vi "PatchViewer.vi"() -> ()   [LabVIEW 2016]
uses:
  <vilib>/Utility/sysdir.llb/System Directory Type.ctl
  <vilib>/Utility/file.llb/Read From Spreadsheet File (DBL).vi
  <vilib>/Utility/file.llb/Write To Spreadsheet File (DBL).vi
  <vilib>/vision/NI_Vision_Development_Module.lvlib
  <vilib>/ptbypt/NI_PtbyPt.lvlib
panel:
  in  "Diff":dbl
  in  "REC":bool
  out "all rows":dbl[][](array[numeric])
  in  "Gamma":dbl(slide)=0.5 min=0.5 max=2.0 step=0.1 scale=0.5..2.0
  in  "Contrast":i64(slide) caption="Gain (Raw)" min=0 max=384 step=1 scale=0.0..100.0
  in  "AutoContrast":bool
  in  "AutoExposure":bool
  in  "Decrease":bool
  in  "Increase":bool
  in  "set 4":bool
  in  "set 3":bool
  in  "set 2":bool
  in  "set 1":bool
  in  "pos 4":bool
  in  "pos 3":bool
  in  "pos 2":bool
  in  "pos 1":bool
  in  "zoom 4":bool
  in  "zoom 3":bool
  in  "zoom 2":bool
  in  "zoom1":bool
  out "fps":dbl
  in  "stop":bool
  in  "Gain":dbl(slide)=1.0 min=1.0 max=4.0 scale=1.0..4.0
  in  "Exposure Time (ms)":dbl(slide)=32000.0 caption="Exposure Time" min=2000.0 max=32000.0 scale=2000.0..32000.0 scale format="%^#_3g"
  out "Image Out":T1(plugin-control)
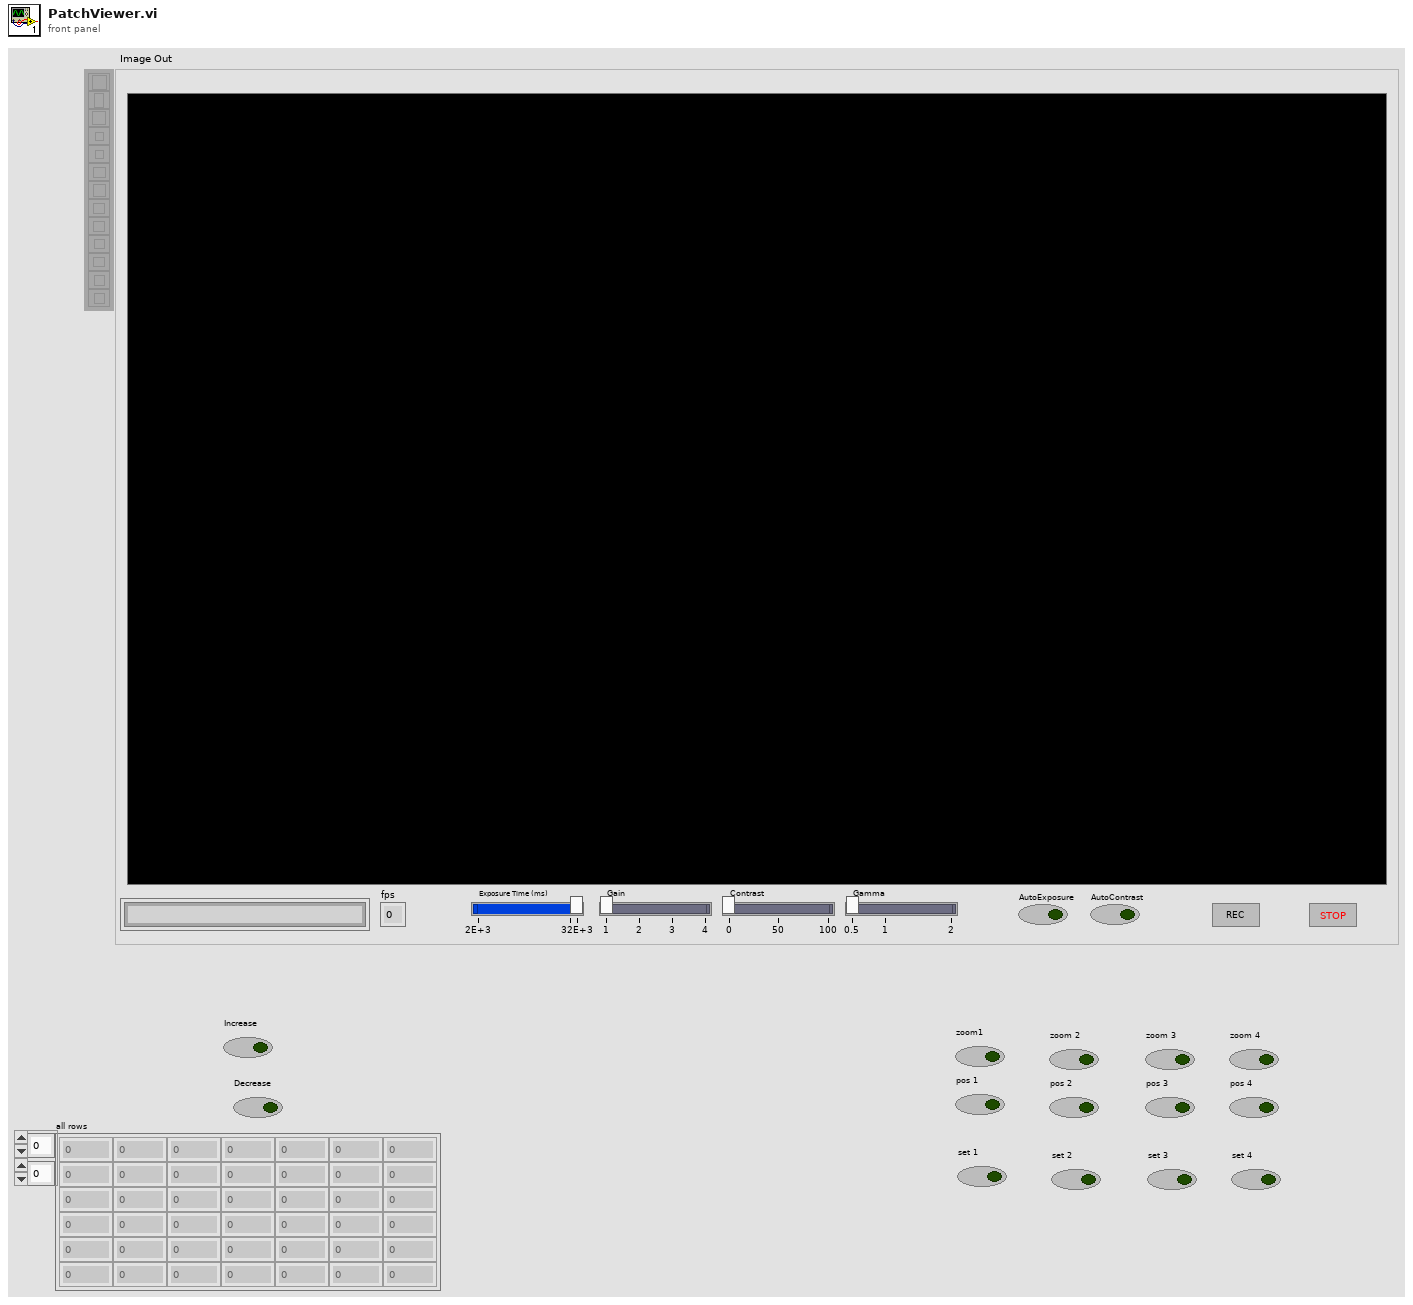
[diagram p1: front panel]
types:
  T1 = typedef "IMAQ Image.ctl" = refnum<image>
  T2 = cluster{"Brightness":sgl, "Contrast":sgl, "Gamma":sgl}
  T3 = cluster{"Mean Value":sgl, "Standard Variation":sgl, "Minimal Value":sgl, "Maximal Value":sgl, "Area (calibrated)":sgl, "Area (pixels)":u32, "%":sgl, "Calibration Valid":bool}
  T4 = typedef "System Directory Type.ctl" = i32
  T5 = typedef "IMAQ AVI2 Refnum.ctl" = refnum<k20>
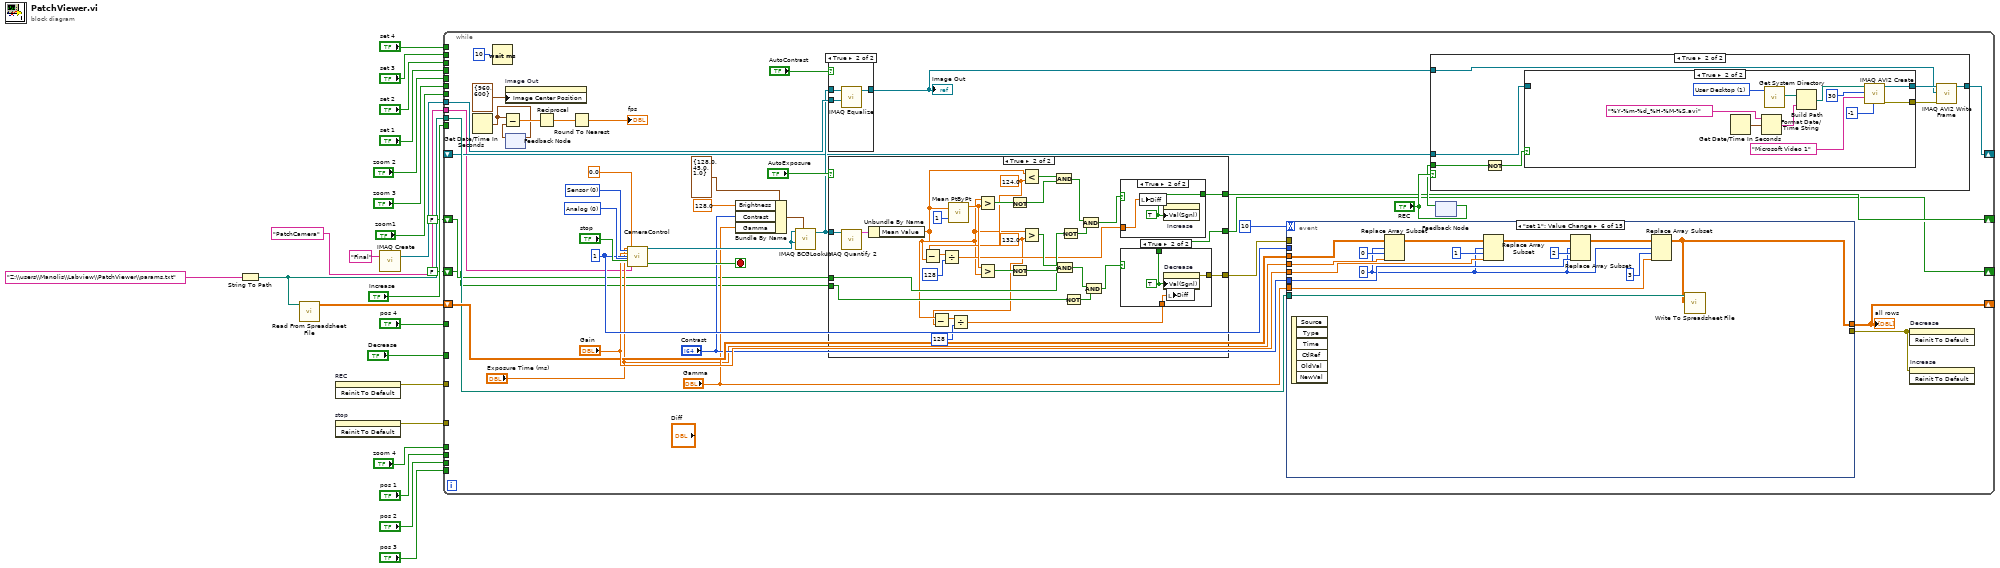
[diagram p0: block diagram]
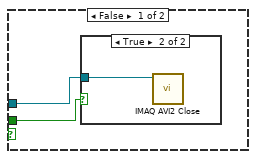
[diagram p2: hidden frame]
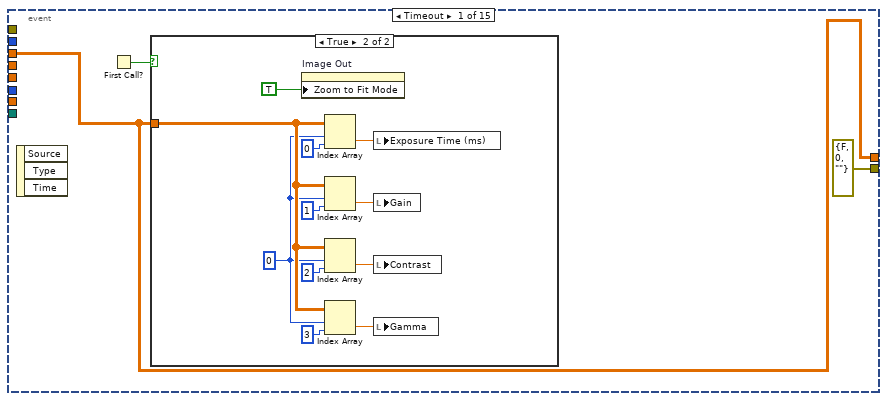
[diagram p9: hidden frame]
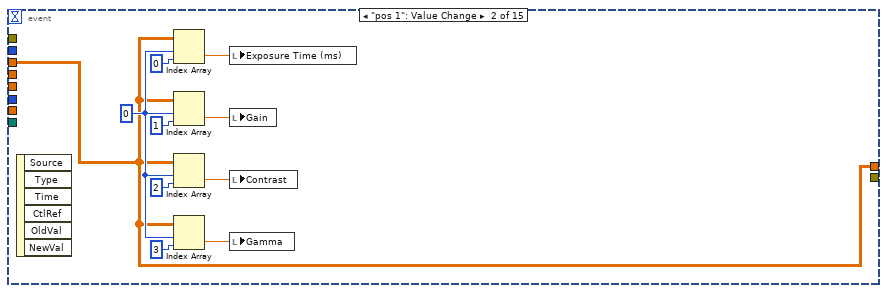
[diagram p11: hidden frame]
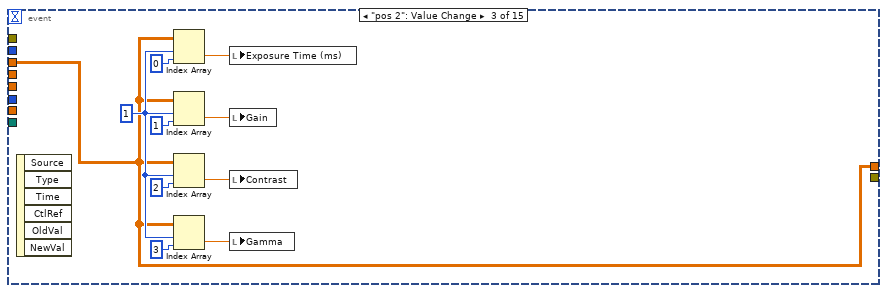
[diagram p12: hidden frame]
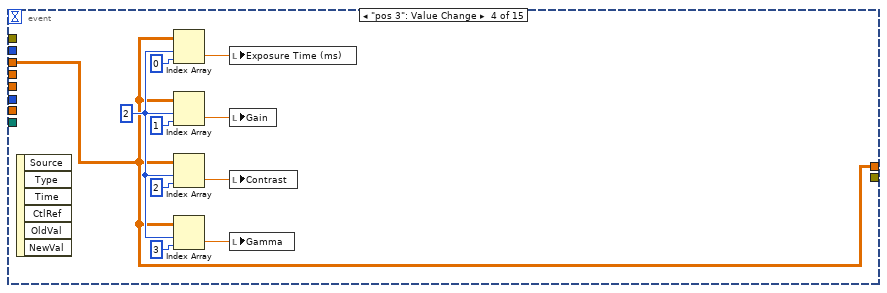
[diagram p13: hidden frame]
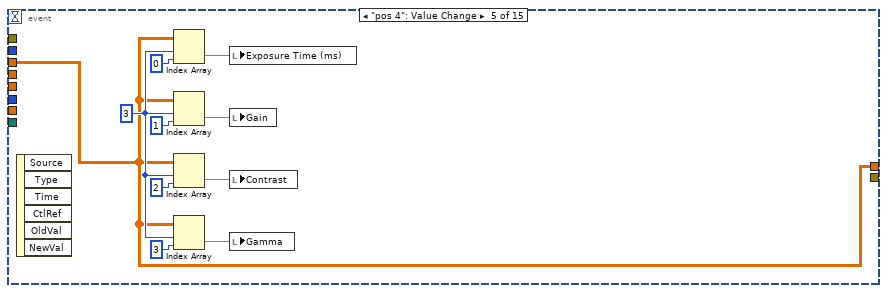
[diagram p14: hidden frame]
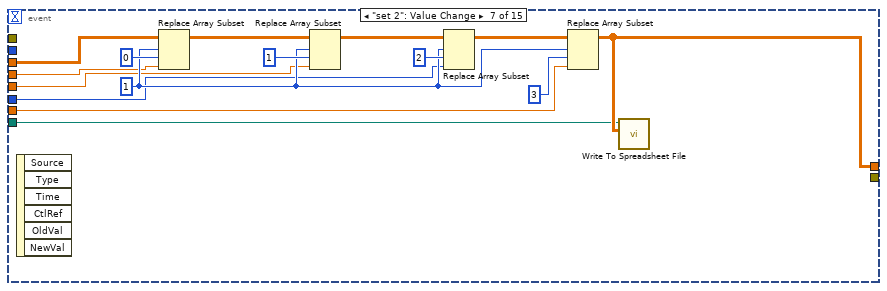
[diagram p15: hidden frame]
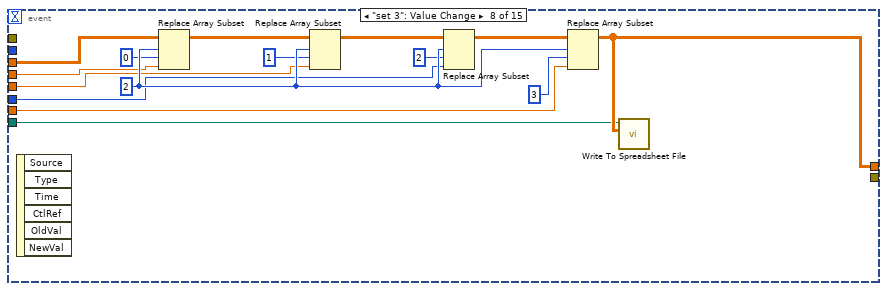
[diagram p16: hidden frame]
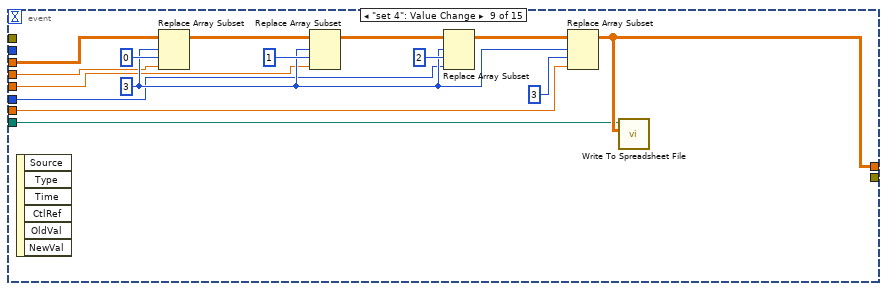
[diagram p17: hidden frame]
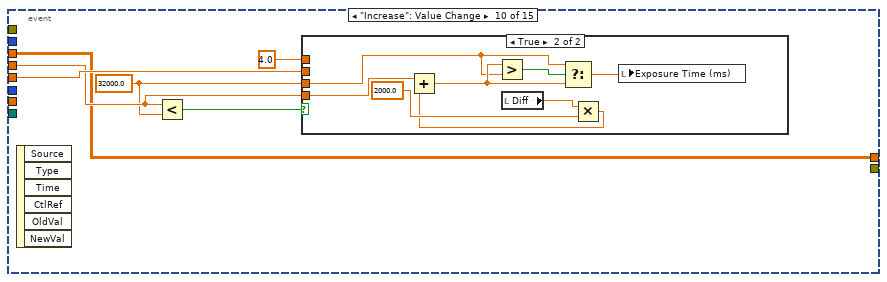
[diagram p18: hidden frame]
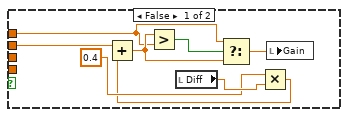
[diagram p19: hidden frame]
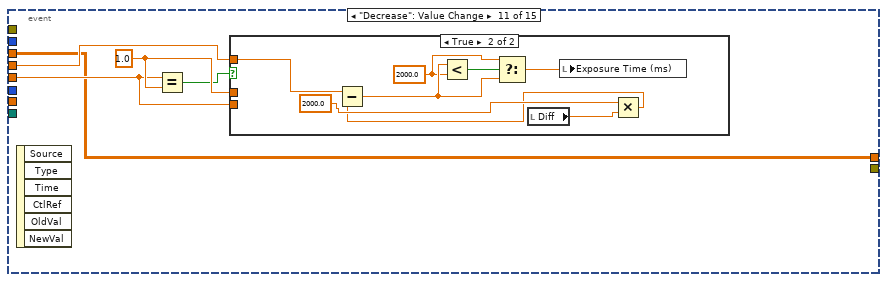
[diagram p20: hidden frame]
diagram:
  n1 = String To Path(string="Z:\\users\\Manolis\\Labview\\PatchViewer\\params.txt") -> (path=w6:path)
  n2 = call-poly <vilib>:"Read From Spreadsheet File.vi"("file path (dialog if empty)"=w6) -> ("all rows"=w7:dbl[][])  [unwired: 6 in, 4 out]
  n3 = invoke on="REC" class="Bool (strict)" method="Reinit To Default"() -> (error out=w5:errorcluster)  [unwired: 3 in, 2 out]
  n4 = invoke on="stop" class="Bool" method="Reinit To Default"() -> (error out=w4:errorcluster)  [unwired: 3 in, 2 out]
  n5 = call "IMAQ Create"("Image Name"="Final") -> ("New Image"=w9:T1)  [unwired: 4 in, 1 out]
  n6 = while {
    tunnel: "pos 4" -> [_]
    tunnel: "pos 3" -> [_]
    tunnel: "pos 2" -> [_]
    tunnel: "pos 1" -> [_]
    tunnel: "zoom1" -> [_]
    tunnel: "zoom 4" -> [_]
    tunnel: "set 4" -> [_]
    tunnel: "set 3" -> [_]
    tunnel: "set 2" -> [_]
    tunnel: "set 1" -> [_]
    tunnel: "zoom 2" -> [_]
    tunnel: "zoom 3" -> [_]
    tunnel: "Increase" -> [_]
    tunnel: "Decrease" -> [_]
    tunnel: w9 -> [w48]
    shift-right: [w45] -> _
    shift-left: w7 -> [w46]
    tunnel: w6 -> [w44]
    shift-right: [w33] -> _
    shift-left: _ -> [w32]
    tunnel: w5 -> [_]
    tunnel: w4 -> [_]
    tunnel: "PatchCamera" -> [w29]
    shift-right: [w28] -> _
    shift-left: FALSE ("Value (Signaling)") -> [w27]
    shift-right: [w26] -> _
    shift-left: FALSE ("Value (Signaling)") -> [w25]
    stop <- w65 stop-if-true
    w53 = i64 1 ("Gain (Raw)")
    w63 = u32 0 items=["Analog"] ("Black Level Selector")
    w64 = u32 0 items=["Sensor", "Digital"] ("Gain Selector")
    n7 = Get Date/Time In Seconds() -> (seconds since 1Jan1904=w59:timestamp)
    n8 = Wait (ms)(milliseconds to wait=u32 10) -> ()  [unwired: 1 out]
    n9 = property on="Image Out" class="ImageControl"("Image Center Position"=cluster{"X":u32, "Y":u32} {"X"=960, "Y"=600} ("Image Center Position:All Elements")) -> ()  [unwired: 2 in, 2 out]
    n10 = feedback-in #1(w59) -> ()
    n11 = feedback #1() -> (w58:timestamp)  [unwired: 1 in]
    n12 = Subtract(x=w59, y=w58) -> (x-y=w60:dbl)
    n13 = Reciprocal(x=w60) -> (1/x=w57:dbl)
    n14 = Round To Nearest(number=w57) -> (nearest integer value=→"fps":dbl)
    n15 = call "CameraControl.vi"("Exposure Time"="Exposure Time (ms)", "Gain Selector"=w64, "Gain"="Gain", "Gain (Raw)"=w53, "Black Level Selector"=w63, "Stop (F)"="stop", "Black Level"=0.0, "Camera"=w29) -> ("Image Out"=w43:T1, "Stopped"=w65:bool)  [unwired: 15 in, 3 out]
    n16 = Bundle By Name(cluster=T2 {"Brightness"=128.0, "Contrast"=45.0, "Gamma"=1.0} ("BCG Values"), "Brightness"=sgl 128.0, "Contrast"="Contrast", "Gamma"="Gamma") -> (w36:T2)
    n17 = call "IMAQ BCGLookup"("Image Src"=w43, "BCG Values"=w36, "Image Dst"=w43) -> ("Image Dst Out"=w41:T1)  [unwired: 4 in, 1 out]
    n18 = case shown="True" "AutoContrast" {
      tunnel: [w88 w90] -> w31
      tunnel: w41 -> [w88 w91]
      tunnel: w48 -> [_ w89]
      frame False {
      }
      frame True {
        n19 = call "IMAQ Equalize"("Image Dst"=w89, "Image Src"=w91) -> ("Image Dst Out"=w90:T1)  [unwired: 8 in, 1 out]
      }
    }
    "Image Out" <- w31
    n20 = case shown="True" "AutoExposure" {
      tunnel: w41 -> [_ w121]
      tunnel: [_ w120] -> w50
      tunnel: [_ w110] -> w28
      tunnel: w27 -> [_ w105]
      tunnel: [_ w109] -> w26
      tunnel: w25 -> [_ w101]
      frame False {
      }
      frame True {
        w100 = sgl 124.0 ("y")
        w93 = sgl 132.0 ("y")
        n21 = call "IMAQ Quantify 2"("Image"=w121) -> ("Global Report"=w111:T3)  [unwired: 8 in, 2 out]
        n22 = Unbundle By Name(w111) -> ("Mean Value"=w94:sgl)
        n23 = Subtract(x=w100, y=w94) -> (x-y=w98:sgl)
        n24 = Subtract(x=w94, y=w93) -> (x-y=w95:sgl)
        n25 = Divide(x=w98, y=128) -> (x/y=w97:sgl)
        n26 = call <vilib>:"Mean PtByPt.vi"("x"=w94, "sample length"=1) -> ("mean"=w113:dbl)  [unwired: 2 in, 1 out]
        n27 = Divide(x=w95, y=128) -> (x/y=w92:sgl)
        n28 = Greater?(x=w94, y=w113) -> (0:w117:bool)
        n29 = Greater?(x=w113, y=w94) -> (0:w114:bool)
        n30 = Not(x=w117) -> (.not. x?=w116:bool)
        n31 = Not(x=w114) -> (.not. x?=w115:bool)
        n32 = Less?(x=w94, y=w100) -> (x < y?=w119:bool)
        n33 = Greater?(x=w94, y=w93) -> (0:w112:bool)
        n34 = And(x=w119, y=w116) -> (x .and. y?=w107:bool)
        n35 = And(x=w112, y=w115) -> (x .and. y?=w102:bool)
        n36 = Not(x=w105) -> (.not. x?=w108:bool)
        n37 = Not(x=w101) -> (.not. x?=w104:bool)
        n38 = And(x=w107, y=w108) -> (x .and. y?=w106:bool)
        n39 = And(x=w102, y=w104) -> (x .and. y?=w103:bool)
        n40 = case shown="True" w106 {
          selector: w106 -> [w122 _]
          tunnel: [w122 w124] -> w110
          tunnel: w97 -> [_ w123]
          frame False {
          }
          frame True {
            w124 = TRUE ("Value (Signaling)")
            n41 = local write "Diff"(w123) -> ()
            n42 = property on="Increase" class="Bool (strict)"("Val(Sgnl)"=w124) -> ()  [unwired: 2 in, 2 out]
          }
        }
        n43 = case shown="True" w103 {
          selector: w103 -> [w125 _]
          tunnel: [_ w128] -> w120
          tunnel: [w125 w127] -> w109
          tunnel: w92 -> [_ w126]
          frame False {
          }
          frame True {
            w127 = TRUE ("Value (Signaling)")
            n44 = property on="Decrease" class="Bool (strict)"("Val(Sgnl)"=w127) -> (error out=w128:errorcluster)  [unwired: 2 in, 1 out]
            n45 = local write "Diff"(w126) -> ()
          }
        }
      }
    }
    n46 = event shown="[5] \"set 1\": Value Change" {
      selector: _ -> [_ _ _ _ _ _ _ _ _ _ _ _ _ _ _]
      dyn-events: _ -> [_ _ _ _ _ _ _ _ _ _ _ _ _ _ _]
      timeout: 10 -> [_ _ _ _ _ _ _ _ _ _ _ _ _ _ _]
      tunnel: "Exposure Time (ms)" -> [_ _ _ _ _ w197 w202 w216 w231 w246 w267 _ _ _ _]
      tunnel: w53 -> [_ _ _ _ _ _ _ _ _ _ _ _ _ _ _]
      tunnel: "Gain" -> [_ _ _ _ _ w196 w201 w215 w230 w248 w268 _ _ _ _]
      tunnel: "Contrast" -> [_ _ _ _ _ w194 w204 w218 w233 _ _ _ _ _ _]
      tunnel: "Gamma" -> [_ _ _ _ _ w193 w203 w217 w232 _ _ _ _ _ _]
      tunnel: [errorcluster {"status"=FALSE, "code"=0, "source"=""} ("error out") _ _ _ _ _ _ _ _ _ _ _ _ _ _] -> w51
      tunnel: w50 -> [_ _ _ _ _ _ _ _ _ _ _ _ _ _ _]
      tunnel: w46 -> [w129 w143 w153 w163 w173 w195 w200 w219 w234 w245 w266 w286 w290 w294 w299]
      tunnel: [w129 w143 w153 w163 w173 w183 w199 w214 w229 w245 w266 w286 w290 w294 w299] -> w45
      tunnel: w44 -> [_ _ _ _ _ w184 w198 w213 w228 _ _ _ _ _ _]
      event Timeout {
        n47 = event-data() -> ()  [unwired: 1 in, 3 out]
        n48 = First Call?() -> (First Call?: T/F=w130:bool)
        n49 = case shown="True" w130 {
          tunnel: w129 -> [_ w141]
          frame False {
          }
          frame True {
            w133 = 0 ("index (row)")
            n50 = property on="Image Out" class="ImageControl"("Zoom to Fit Mode"=TRUE) -> ()  [unwired: 2 in, 2 out]
            n51 = Index Array(array=w141, index (row)=w133, index (col)=0 ("disabled index (col)")) -> (element=w137:dbl)
            n52 = Index Array(array=w141, index (row)=w133, index (col)=1 ("disabled index (col)")) -> (element=w136:dbl)
            n53 = Index Array(array=w141, index (row)=w133, index (col)=2 ("disabled index (col)")) -> (element=w135:dbl)
            n54 = Index Array(array=w141, index (row)=w133, index (col)=3 ("disabled index (col)")) -> (element=w134:dbl)
            n55 = local write "Exposure Time (ms)"(w137) -> ()
            n56 = local write "Gain"(w136) -> ()
            n57 = local write "Contrast"(w135) -> ()
            n58 = local write "Gamma"(w134) -> ()
          }
        }
      }
      event "pos 1": Value Change {
        w152 = 0 ("index (row)")
        n59 = event-data() -> ()  [unwired: 1 in, 6 out]
        n60 = Index Array(array=w143, index (row)=w152, index (col)=0 ("disabled index (col)")) -> (element=w148:dbl)
        n61 = Index Array(array=w143, index (row)=w152, index (col)=1 ("disabled index (col)")) -> (element=w149:dbl)
        n62 = Index Array(array=w143, index (row)=w152, index (col)=2 ("disabled index (col)")) -> (element=w150:dbl)
        n63 = Index Array(array=w143, index (row)=w152, index (col)=3 ("disabled index (col)")) -> (element=w151:dbl)
        n64 = local write "Exposure Time (ms)"(w148) -> ()
        n65 = local write "Gain"(w149) -> ()
        n66 = local write "Contrast"(w150) -> ()
        n67 = local write "Gamma"(w151) -> ()
      }
      event "pos 2": Value Change {
        w154 = 1 ("index (row)")
        n68 = event-data() -> ()  [unwired: 1 in, 6 out]
        n69 = Index Array(array=w153, index (row)=w154, index (col)=0 ("disabled index (col)")) -> (element=w158:dbl)
        n70 = Index Array(array=w153, index (row)=w154, index (col)=1 ("disabled index (col)")) -> (element=w157:dbl)
        n71 = Index Array(array=w153, index (row)=w154, index (col)=2 ("disabled index (col)")) -> (element=w156:dbl)
        n72 = Index Array(array=w153, index (row)=w154, index (col)=3 ("disabled index (col)")) -> (element=w155:dbl)
        n73 = local write "Exposure Time (ms)"(w158) -> ()
        n74 = local write "Gain"(w157) -> ()
        n75 = local write "Contrast"(w156) -> ()
        n76 = local write "Gamma"(w155) -> ()
      }
      event "pos 3": Value Change {
        w172 = 2 ("index (row)")
        n77 = event-data() -> ()  [unwired: 1 in, 6 out]
        n78 = Index Array(array=w163, index (row)=w172, index (col)=0 ("disabled index (col)")) -> (element=w168:dbl)
        n79 = Index Array(array=w163, index (row)=w172, index (col)=1 ("disabled index (col)")) -> (element=w169:dbl)
        n80 = Index Array(array=w163, index (row)=w172, index (col)=2 ("disabled index (col)")) -> (element=w170:dbl)
        n81 = Index Array(array=w163, index (row)=w172, index (col)=3 ("disabled index (col)")) -> (element=w171:dbl)
        n82 = local write "Exposure Time (ms)"(w168) -> ()
        n83 = local write "Gain"(w169) -> ()
        n84 = local write "Contrast"(w170) -> ()
        n85 = local write "Gamma"(w171) -> ()
      }
      event "pos 4": Value Change {
        w174 = 3 ("index (row)")
        n86 = event-data() -> ()  [unwired: 1 in, 6 out]
        n87 = Index Array(array=w173, index (row)=w174, index (col)=0 ("disabled index (col)")) -> (element=w178:dbl)
        n88 = Index Array(array=w173, index (row)=w174, index (col)=1 ("disabled index (col)")) -> (element=w177:dbl)
        n89 = Index Array(array=w173, index (row)=w174, index (col)=2 ("disabled index (col)")) -> (element=w176:dbl)
        n90 = Index Array(array=w173, index (row)=w174, index (col)=3 ("disabled index (col)")) -> (element=w175:dbl)
        n91 = local write "Exposure Time (ms)"(w178) -> ()
        n92 = local write "Gain"(w177) -> ()
        n93 = local write "Contrast"(w176) -> ()
        n94 = local write "Gamma"(w175) -> ()
      }
      event "set 1": Value Change {
        w185 = 0 ("index (row)")
        n95 = event-data() -> ()  [unwired: 1 in, 6 out]
        n96 = Replace Array Subset(array=w195, new element=w197, index (row)=w185, index (col)=0 ("index (row)")) -> (w192:dbl[][])
        n97 = Replace Array Subset(array=w192, new element=w196, index (row)=w185, index (col)=1 ("index (row)")) -> (w191:dbl[][])
        n98 = Replace Array Subset(array=w191, new element=w194, index (row)=w185, index (col)=2 ("index (row)")) -> (w190:dbl[][])
        n99 = Replace Array Subset(array=w190, new element=w193, index (row)=w185, index (col)=3 ("index (row)")) -> (w183:dbl[][])
        n100 = call-poly <vilib>:"Write To Spreadsheet File.vi"("2D data"=w183, "file path (dialog if empty)"=w184) -> ()  [unwired: 6 in, 1 out]
      }
      event "set 2": Value Change {
        w205 = 1 ("index (row)")
        n101 = event-data() -> ()  [unwired: 1 in, 6 out]
        n102 = Replace Array Subset(array=w200, new element=w202, index (row)=w205, index (col)=0 ("index (row)")) -> (w212:dbl[][])
        n103 = Replace Array Subset(array=w212, new element=w201, index (row)=w205, index (col)=1 ("index (row)")) -> (w211:dbl[][])
        n104 = Replace Array Subset(array=w211, new element=w204, index (row)=w205, index (col)=2 ("index (row)")) -> (w210:dbl[][])
        n105 = Replace Array Subset(array=w210, new element=w203, index (row)=w205, index (col)=3 ("index (row)")) -> (w199:dbl[][])
        n106 = call-poly <vilib>:"Write To Spreadsheet File.vi"("2D data"=w199, "file path (dialog if empty)"=w198) -> ()  [unwired: 6 in, 1 out]
      }
      event "set 3": Value Change {
        w227 = 2 ("index (row)")
        n107 = event-data() -> ()  [unwired: 1 in, 6 out]
        n108 = Replace Array Subset(array=w219, new element=w216, index (row)=w227, index (col)=0 ("index (row)")) -> (w220:dbl[][])
        n109 = Replace Array Subset(array=w220, new element=w215, index (row)=w227, index (col)=1 ("index (row)")) -> (w221:dbl[][])
        n110 = Replace Array Subset(array=w221, new element=w218, index (row)=w227, index (col)=2 ("index (row)")) -> (w222:dbl[][])
        n111 = Replace Array Subset(array=w222, new element=w217, index (row)=w227, index (col)=3 ("index (row)")) -> (w214:dbl[][])
        n112 = call-poly <vilib>:"Write To Spreadsheet File.vi"("2D data"=w214, "file path (dialog if empty)"=w213) -> ()  [unwired: 6 in, 1 out]
      }
      event "set 4": Value Change {
        w235 = 3 ("index (row)")
        n113 = event-data() -> ()  [unwired: 1 in, 6 out]
        n114 = Replace Array Subset(array=w234, new element=w231, index (row)=w235, index (col)=0 ("index (row)")) -> (w242:dbl[][])
        n115 = Replace Array Subset(array=w242, new element=w230, index (row)=w235, index (col)=1 ("index (row)")) -> (w241:dbl[][])
        n116 = Replace Array Subset(array=w241, new element=w233, index (row)=w235, index (col)=2 ("index (row)")) -> (w240:dbl[][])
        n117 = Replace Array Subset(array=w240, new element=w232, index (row)=w235, index (col)=3 ("index (row)")) -> (w229:dbl[][])
        n118 = call-poly <vilib>:"Write To Spreadsheet File.vi"("2D data"=w229, "file path (dialog if empty)"=w228) -> ()  [unwired: 6 in, 1 out]
      }
      event "Increase": Value Change {
        w243 = 32000.0 ("y")
        n119 = event-data() -> ()  [unwired: 1 in, 6 out]
        n120 = Less?(x=w246, y=w243) -> (x < y?=w244:bool)
        n121 = case shown="True" w244 {
          tunnel: w246 -> [_ w264]
          tunnel: w248 -> [w256 _]
          tunnel: 4.0 ("y") -> [w252 _]
          tunnel: w243 -> [_ w260]
          frame False {
            n122 = local read "Diff"() -> (w251:dbl)
            n123 = Multiply(x=0.4 ("y"), y=w251) -> (x*y=w249:dbl)
            n124 = Add(x=w256, y=w249) -> (x+y=w254:dbl)
            n125 = Greater?(x=w254, y=w252) -> (0:w255:bool)
            n126 = Select(t=w252, s=w255, f=w254) -> (s? t:f=w253:dbl)
            n127 = local write "Gain"(w253) -> ()
          }
          frame True {
            n128 = local read "Diff"() -> (w259:dbl)
            n129 = Multiply(x=w259, y=2000.0) -> (x*y=w257:dbl)
            n130 = Add(x=w264, y=w257) -> (x+y=w262:dbl)
            n131 = Greater?(x=w262, y=w260) -> (0:w263:bool)
            n132 = Select(t=w260, s=w263, f=w262) -> (s? t:f=w261:dbl)
            n133 = local write "Exposure Time (ms)"(w261) -> ()
          }
        }
      }
      event "Decrease": Value Change {
        w269 = 1.0 ("y")
        n134 = event-data() -> ()  [unwired: 1 in, 6 out]
        n135 = Equal?(x=w268, y=w269) -> (x = y?=w265:bool)
        n136 = case shown="True" w265 {
          tunnel: w267 -> [_ w285]
          tunnel: w268 -> [w277 _]
          tunnel: w269 -> [w273 _]
          frame False {
            n137 = local read "Diff"() -> (w272:dbl)
            n138 = Multiply(x=0.4 ("y"), y=w272) -> (x*y=w270:dbl)
            n139 = Subtract(x=w277, y=w270) -> (x-y=w275:dbl)
            n140 = Less?(x=w275, y=w273) -> (x < y?=w276:bool)
            n141 = Select(t=w273, s=w276, f=w275) -> (s? t:f=w274:dbl)
            n142 = local write "Gain"(w274) -> ()
          }
          frame True {
            w282 = 2000.0 ("y")
            n143 = local read "Diff"() -> (w280:dbl)
            n144 = Multiply(x=2000.0 ("y"), y=w280) -> (x*y=w278:dbl)
            n145 = Subtract(x=w285, y=w278) -> (x-y=w283:dbl)
            n146 = Less?(x=w283, y=w282) -> (x < y?=w284:bool)
            n147 = Select(t=w282, s=w284, f=w283) -> (s? t:f=w281:dbl)
            n148 = local write "Exposure Time (ms)"(w281) -> ()
          }
        }
      }
      event "zoom1": Value Change {
        n149 = event-data() -> ()  [unwired: 1 in, 6 out]
        n150 = property on="Image Out" class="ImageControl"("Zoom to Fit Mode"=TRUE) -> ()  [unwired: 2 in, 2 out]
      }
      event "zoom 2": Value Change {
        w288 = 0.75
        n151 = event-data() -> ()  [unwired: 1 in, 6 out]
        n152 = Bundle By Name(cluster=cluster{"X":sgl, "Y":sgl} {"X"=0.0, "Y"=0.0} ("ZoomSingle:All Elements"), "X"=w288, "Y"=w288) -> (w291:cluster{"X":sgl, "Y":sgl})
        n153 = property on="Image Out" class="ImageControl"("ZoomSingle"=w291) -> ()  [unwired: 2 in, 2 out]
      }
      event "zoom 3": Value Change {
        w292 = 1.0
        n154 = event-data() -> ()  [unwired: 1 in, 6 out]
        n155 = Bundle By Name(cluster=cluster{"X":sgl, "Y":sgl} {"X"=0.0, "Y"=0.0} ("ZoomSingle:All Elements"), "X"=w292, "Y"=w292) -> (w295:cluster{"X":sgl, "Y":sgl})
        n156 = flat-sequence {
          tunnel: w295 -> [w296]
          frame #0 {
            n157 = property on="Image Out" class="ImageControl"("ZoomSingle"=w296) -> ()  [unwired: 2 in, 2 out]
          }
        }
      }
      event "zoom 4": Value Change {
        w297 = 1.5
        n158 = event-data() -> ()  [unwired: 1 in, 6 out]
        n159 = Bundle By Name(cluster=cluster{"X":sgl, "Y":sgl} {"X"=0.0, "Y"=0.0} ("ZoomSingle:All Elements"), "X"=w297, "Y"=w297) -> (w300:cluster{"X":sgl, "Y":sgl})
        n160 = flat-sequence {
          tunnel: w300 -> [w301]
          frame #0 {
            n161 = property on="Image Out" class="ImageControl"("ZoomSingle"=w301) -> ()  [unwired: 2 in, 2 out]
          }
        }
      }
    }
    "all rows" <- w45
    n162 = feedback #2() -> (w34:bool)  [unwired: 1 in]
    n163 = case shown="True" "REC" {
      tunnel: w31 -> [_ w73]
      tunnel: [_ w72] -> w33
      tunnel: w32 -> [w67 w71]
      tunnel: w34 -> [w66 w69]
      frame False {
        n164 = case shown="True" w66 {
          tunnel: w67 -> [_ w68]
          frame False {
          }
          frame True {
            n165 = call "IMAQ AVI2 Close"("AVI Refnum"=w68) -> ()  [unwired: 10 in, 1 out]
          }
        }
      }
      frame True {
        n166 = Not(x=w69) -> (.not. x?=w70:bool)
        n167 = case shown="True" w70 {
          tunnel: [w76 w87] -> w75
          tunnel: [_ w83] -> w74
          tunnel: w71 -> [w76 _]
          frame False {
          }
          frame True {
            w78 = T4 1 items=["User Home"=0, "User Desktop"=1, "User Documents"=2, "User Application Data"=3, "User Preferences"=4, "User Temporary"=5, "Public Documents"=6, "Public Application Data"=7, "Public Preferences"=8, "Public Cache"=13, "System Core Libraries"=9, "System Installed Libraries"=10, "Application Files"=11, "Boot Volume Root"=12] ("system directory type")
            n168 = Get Date/Time In Seconds() -> (seconds since 1Jan1904=w81:timestamp)
            n169 = Format Date/Time String(time format string (%c)="%Y-%m-%d_%H-%M-%S.avi", seconds (now)=w81) -> (date/time string=w82:string)  [unwired: 1 out]
            n170 = call <vilib>:"Get System Directory.vi"("system directory type"=w78) -> ("system directory"=w77:path)  [unwired: 10 in]
            n171 = Build Path(base path=w77, name or relative path=w82) -> (appended path=w79:path)
            n172 = call "IMAQ AVI2 Create"("Quality"=-1, "Codec"="Microsoft Video 1", "Frames Per Second"=u32 30, "AVI Path"=w79) -> ("error out"=w83:errorcluster, "AVI Refnum"=w87:T5)  [unwired: 6 in]
          }
        }
        n173 = call "IMAQ AVI2 Write Frame"("error in (no error)"=w74, "Image"=w73, "AVI Refnum"=w75) -> ("AVI Refnum (duplicate)"=w72:T5)  [unwired: 6 in, 2 out]
      }
    }
    n174 = feedback-in #2("REC") -> ()
    n175 = invoke on="Decrease" class="Bool (strict)" method="Reinit To Default"(error in=w51) -> ()  [unwired: 2 in, 3 out]
    n176 = invoke on="Increase" class="Bool (strict)" method="Reinit To Default"(error in=w51) -> ()  [unwired: 2 in, 3 out]
  }
